vi "myPICO_Close.vi"(6 "数值":u16, 10 "数组":T2(array[cluster])) -> ()   [LabVIEW 2024]
uses:
  shared/PicoBuffers.ctl
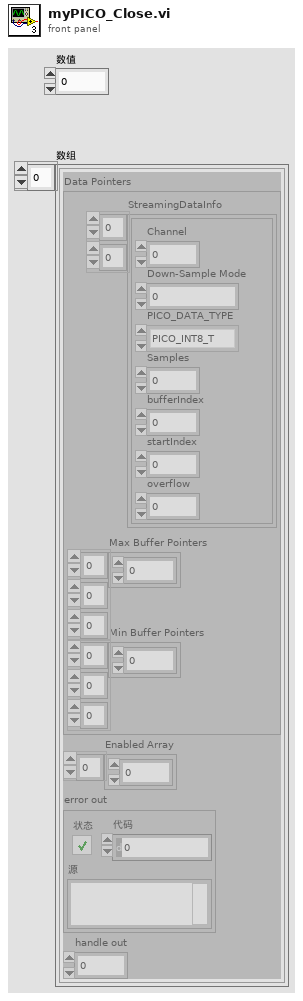
[diagram p1: front panel]
types:
  T1 = typedef "PicoBuffers.ctl" = cluster{"Max Buffer Pointers":u64[][][], "Min Buffer Pointers":u64[][][], "StreamingDataInfo":cluster{"Channel":u32, "Down-Sample Mode":u32, "PICO_DATA_TYPE":enum32{"PICO_INT8_T", "PICO_INT16_T", "PICO_INT32_T", "PICO_UINT32_T", "PICO_INT64_T", ""}, "Samples":i32, "bufferIndex":u64, "startIndex":i32, "overflow":i16}[][]}
  T2 = cluster{"Data Pointers":T1, "Enabled Array":i16[], "error out":errorcluster, "handle out":i16}[]
  T3 = cluster{"Data Pointers":T1, "Enabled Array":i16[], "error out":errorcluster, "handle out":i16}
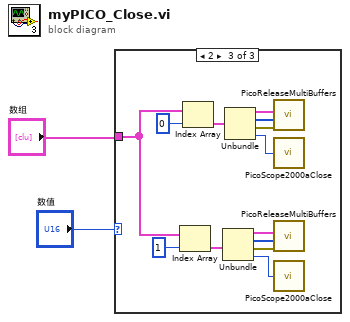
[diagram p0: block diagram]
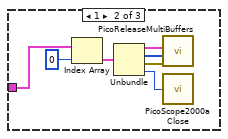
[diagram p3: hidden frame]
diagram:
  n1 = case shown="2" "数值" {
    tunnel: "数组" -> [_ w3 w10]
    frame 0, Default {
    }
    frame 1 {
      n2 = Index Array(array=w3, index=0 ("索引")) -> (element=w9:T3)
      n3 = Unbundle(w9) -> ("Data Pointers"=w8:T1, "Enabled Array"=w7:i16[], "error out"=w6:errorcluster, "handle out"=w5:i16)
      n4 = call "PicoReleaseMultiBuffers.vi"("error in (no error)"=w6, "Enabled array"=w7, "Data Pointers"=w8) -> ()  [unwired: 8 in, 1 out]
      n5 = call "PicoScope2000aClose.vi"("handle"=w5) -> ()
    }
    frame 2 {
      n6 = Index Array(array=w10, index=1 ("索引")) -> (element=w21:T3)
      n7 = Index Array(array=w10, index=0 ("索引")) -> (element=w16:T3)
      n8 = Unbundle(w21) -> ("Data Pointers"=w20:T1, "Enabled Array"=w19:i16[], "error out"=w18:errorcluster, "handle out"=w17:i16)
      n9 = Unbundle(w16) -> ("Data Pointers"=w15:T1, "Enabled Array"=w14:i16[], "error out"=w13:errorcluster, "handle out"=w12:i16)
      n10 = call "PicoReleaseMultiBuffers.vi"("error in (no error)"=w13, "Enabled array"=w14, "Data Pointers"=w15) -> ()  [unwired: 8 in, 1 out]
      n11 = call "PicoScope2000aClose.vi"("handle"=w12) -> ()
      n12 = call "PicoReleaseMultiBuffers.vi"("error in (no error)"=w18, "Enabled array"=w19, "Data Pointers"=w20) -> ()  [unwired: 8 in, 1 out]
      n13 = call "PicoScope2000aClose.vi"("handle"=w17) -> ()
    }
  }
